vi "6343test.vi"() -> ()   [LabVIEW 2013]
panel:
  in  "数组":dbl[](array[numeric])
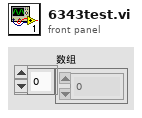
[diagram p1: front panel]
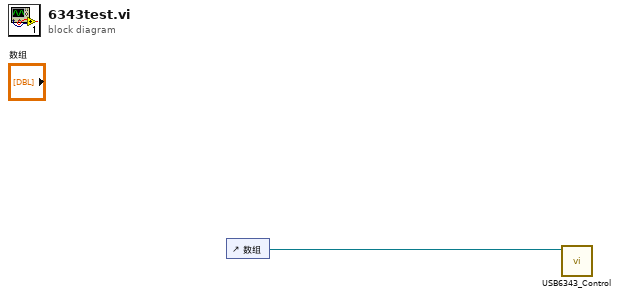
[diagram p0: block diagram]
diagram:
  n1 = control-ref of="数组"() -> (w1:refnum<vi>)
  n2 = call "USB6343_Control.vi"("monitor buff"=w1) -> ()  [unwired: 9 in, 2 out]
